vi "Write States.vi"(8 "error in (no error)":errorcluster, 10 "States":enum16{"Exit", "FollowAttacker"}(ring), 11 "FollowAttackerTactic in":refnum<class "FollowAttackerTactic.lvclass">) -> (0 "error out":errorcluster, 3 "FollowAttackerTactic out":refnum<class "FollowAttackerTactic.lvclass">)   [LabVIEW 2020, in "FollowAttackerTactic.lvclass"]
uses:
  FollowAttackerTactic.lvclass
  FollowAttackerTactic.lvclass/FollowAttackerTactic.ctl
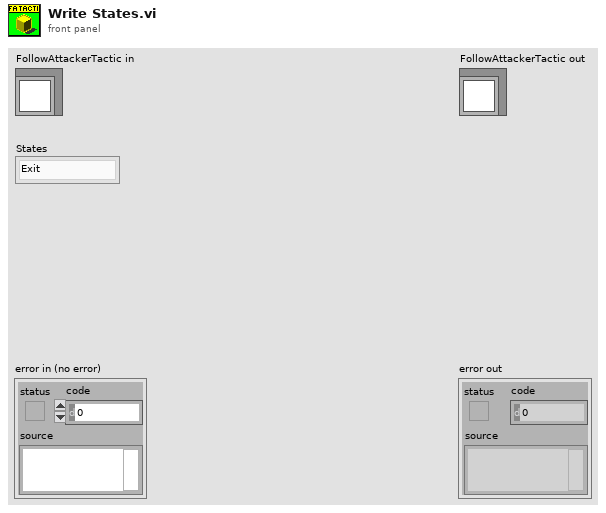
[diagram p1: front panel]
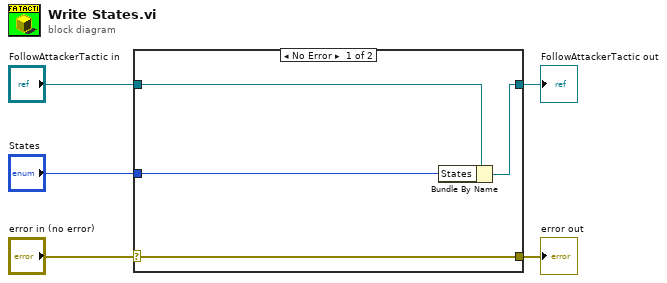
[diagram p0: block diagram]
diagram:
  n1 = case shown="No Error" "error in (no error)" {
    selector: "error in (no error)" -> [w9 w10]
    tunnel: [w9 w10] -> w4
    tunnel: [w7 w11] -> w2
    tunnel: "FollowAttackerTactic in" -> [w8 w11]
    tunnel: "States" -> [w6 _]
    frame No Error {
      n2 = Bundle By Name(cluster=w8, "States"=w6) -> (w7:refnum<class "FollowAttackerTactic.lvclass">)
    }
    frame Error {
    }
  }
  "error out" <- w4
  "FollowAttackerTactic out" <- w2
